vi "DS402 Drive - Get Slave Data.vi"(8 "error in (no error)":errorcluster caption="Fehler (Eingang, kein Fehler)", 11 "EtherCAT Slave In":T10 {"VS ref" format="%.0x"}) -> (0 "error out":errorcluster caption="Fehler (Ausgang)", 3 "EtherCAT Slave out":T1 {"I/O Output Data"."BD Refs"."Data Reference" format="%.0x"; "I/O Input Data"."BD Refs"."Data Reference" format="%.0x"; "I/O Output Vars"."VS ref" format="%.0x"; "I/O Input Vars"."VS ref" format="%.0x"; "VS ref" format="%.0x"})   [LabVIEW 2016, in "Scan Engine Custom Device.lvlib"]
uses:
  Scan Engine Custom Device.lvlib
  <vilib>/NI Veristand/Custom Device API/Custom Device Item Ref.ctl
  Type Defs/DS402 Drive ECAT Slave Data Cluster.ctl
  Type Defs/DS402 Drive ECAT Slave IOV Cluster.ctl
  Type Defs/UDV Data Type.ctl
  Type Defs/Input Data.ctl
  <vilib>/NI Veristand/Custom Device API/Block Data Reference.ctl
  <vilib>/NI Veristand/Custom Device API/Data Reference.ctl
  Type Defs/Output Data.ctl
  Type Defs/DS402 Drive ECAT Slave Action IOV Cluster.ctl
  <vilib>/NI Veristand/Custom Device API/Get Item Property (I32).vi
  Globals/Property Strings.vi
  <vilib>/NI Veristand/Custom Device API/Custom Device API.lvlib
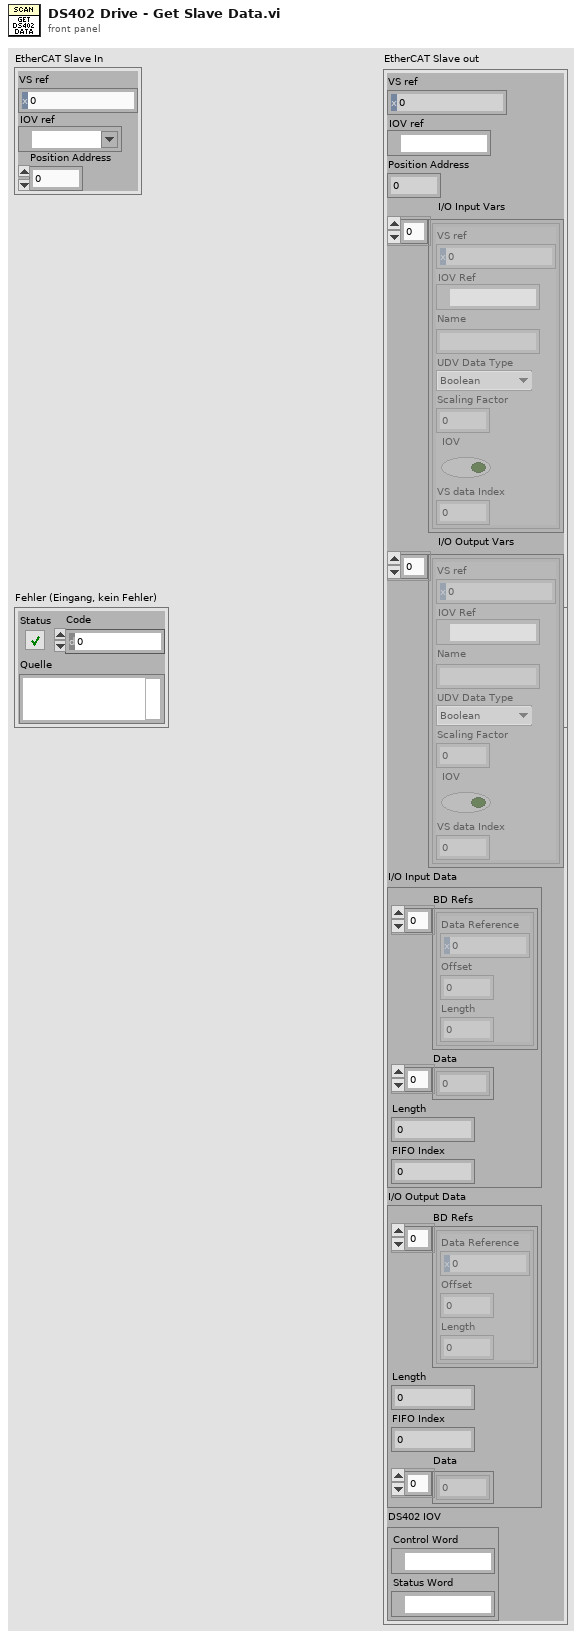
[diagram p1: front panel]
types:
  T1 = typedef "Scan Engine Custom Device.lvlib/DS402 Drive ECAT Slave Data Cluster.ctl" = cluster{"VS ref":T2, "IOV ref":refnum<k21>, "Position Address":u16, "I/O Input Vars ":T3[], "I/O Output Vars":T3[], "I/O Input Data":T5, "I/O Output Data":T8, "DS402 IOV":T9}
  T2 = typedef "Custom Device API.lvlib/Custom Device Item Ref.ctl" = u64
  T3 = typedef "Scan Engine Custom Device.lvlib/DS402 Drive ECAT Slave IOV Cluster.ctl" = cluster{"VS ref":T2, "IOV Ref":refnum<k21>, "Name":string, "UDV Data Type":T4, "Scaling Factor":dbl, "IOV":bool, "VS data Index":i32}
  T4 = typedef "Scan Engine Custom Device.lvlib/UDV Data Type.ctl" = enum16{"Boolean", "Fixed Point", "Int8", "Int16", "Int32", "Int64", "U32 Bit Field", "UInt8", "UInt16", "UInt32", "UInt64", "Other"}
  T5 = typedef "Scan Engine Custom Device.lvlib/Input Data.ctl" = cluster{"BD Refs":T6[], "Data":dbl[], "Length":i32, "FIFO Index":i32}
  T6 = typedef "Custom Device API.lvlib/Block Data Reference.ctl" = cluster{"Data Reference":T7, "Offset":u64, "Length":u64}
  T7 = typedef "Custom Device API.lvlib/Data Reference.ctl" = i32
  T8 = typedef "Scan Engine Custom Device.lvlib/Output Data.ctl" = cluster{"BD Refs":T6[], "Length":i32, "FIFO Index":i32, "Data":dbl[]}
  T9 = typedef "Scan Engine Custom Device.lvlib/DS402 Drive ECAT Slave Action IOV Cluster.ctl" = cluster{"Control Word":refnum<k21>, "Status Word":refnum<k21>}
  T10 = cluster{"VS ref":T2, "IOV ref":refnum<k21>, "Position Address":u16}
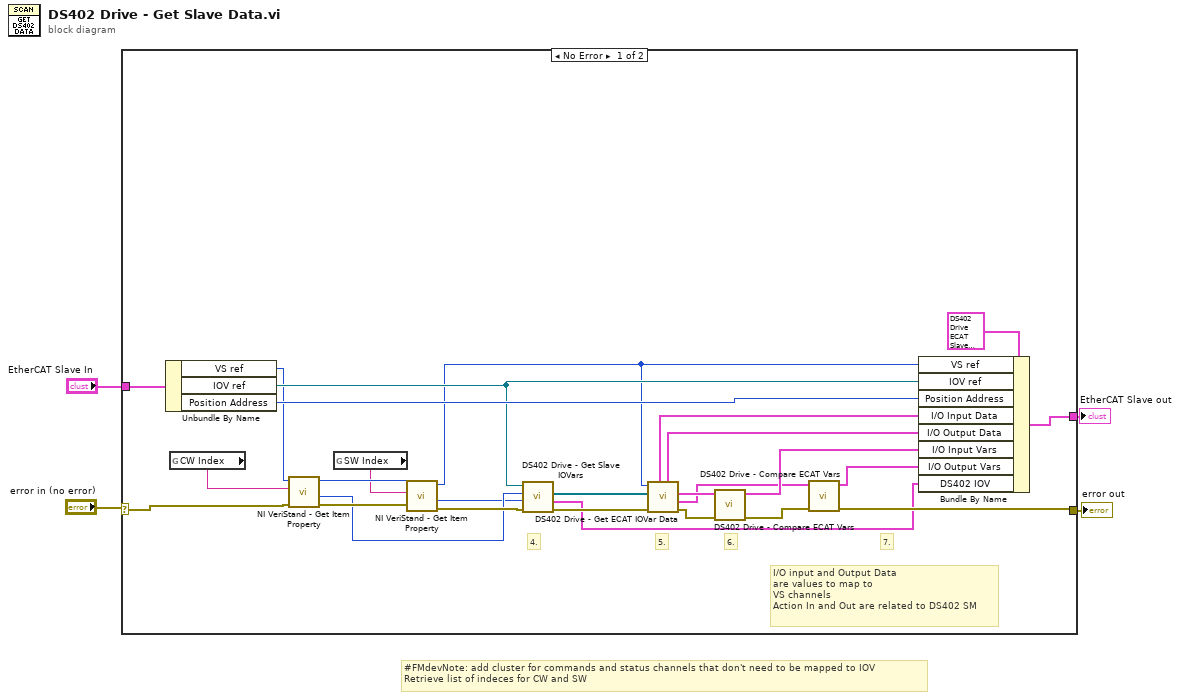
[diagram p0: block diagram]
diagram:
  # "#FMdevNote: add cluster for commands and status channels that don't need to be mapped to IOV\nRetrieve list of indeces for CW and SW"
  n1 = case shown="No Error" "error in (no error)" {
    selector: "error in (no error)" -> [w9 w32]
    tunnel: "EtherCAT Slave In" -> [w30 _]
    tunnel: [w24 w32] -> w2
    tunnel: [w28 _] -> w1
    frame No Error {
      # "I/O input and Output Data\nare values to map to \nVS channels\nAction In and Out are related to DS402 SM"
      # "7."
      # "6."
      # "5."
      # "4."
      n2 = Unbundle By Name(w30) -> ("VS ref"=w14:T2, "IOV ref"=w15:refnum<k21>, "Position Address"=w29:u16)
      n3 = global read "Property Strings.vi" "CW Index"() -> (w8:string)
      n4 = call-poly <vilib>:"NI VeriStand - Get Item Property.vi"("error in (no error)"=w9, "Property Name"=w8, "Item Ref in"=w14) -> ("error out"=w11:errorcluster, "Value"=w6:i32, "Item Ref out"=w13:T2)  [unwired: 5 in, 1 out]
      n5 = global read "Property Strings.vi" "SW Index"() -> (w7:string)
      n6 = call-poly <vilib>:"NI VeriStand - Get Item Property.vi"("error in (no error)"=w11, "Property Name"=w7, "Item Ref in"=w13) -> ("error out"=w10:errorcluster, "Value"=w5:i32, "Item Ref out"=w12:T2)  [unwired: 5 in, 1 out]
      n7 = call "DS402 Drive - Get Slave IOVars.vi"("error in (no error)"=w10, "SW Index"=w5, "CW Index"=w6, "ECAT Slave in"=w15) -> ("error IO"=w27:errorcluster, "DS402 IOV"=w16:T9, "ECAT IO Variables"=w17:refnum<k21>[])  [unwired: 3 in, 2 out]
      n8 = call "DS402 Drive - Get ECAT IOVar Data.vi"("error in (no error)"=w27, "ECAT IO Variable In"=w17, "VS ref"=w12) -> ("Error out"=w26:errorcluster, "I/O Output Vars"=w18:T3[], "I/O Input Vars"=w21:T3[], "I/O Output Data"=w22:T8, "I/O Input Data"=w23:T5)  [unwired: 3 in, 1 out]
      n9 = call "DS402 Drive - Compare ECAT Vars.vi"("Fehler (Eingang, kein Fehler)"=w26, "I/O Vars In"=w21) -> ("Fehler (Ausgang)"=w25:errorcluster, "I/O Vars Out"=w20:T3[])  [unwired: 8 in]
      n10 = call "DS402 Drive - Compare ECAT Vars.vi"("Fehler (Eingang, kein Fehler)"=w25, "I/O Vars In"=w18) -> ("Fehler (Ausgang)"=w24:errorcluster, "I/O Vars Out"=w19:T3[])  [unwired: 8 in]
      n11 = Bundle By Name(cluster=T1 {"VS ref"=0, "IOV ref"="", "Position Address"=0, "I/O Input Vars "=[], "I/O Output Vars"=[], "I/O Input Data"={"BD Refs"=[], "Data"=[], "Length"=0, "FIFO Index"=0}, "I/O Output Data"={"BD Refs"=[], "Length"=0, "FIFO Index"=0, "Data"=[]}, "DS402 IOV"={"Control Word"="", "Status Word"=""}} ("EtherCAT Slave"), "VS ref"=w12, "IOV ref"=w15, "Position Address"=w29, "I/O Input Data"=w23, "I/O Output Data"=w22, "I/O Input Vars"=w20, "I/O Output Vars"=w19, "DS402 IOV"=w16) -> (w28:T1)
    }
    frame Error {
    }
  }
  "error out" <- w2
  "EtherCAT Slave out" <- w1
